vi "Subvi Add Offset to XY Coordinates.vi"(1 "YOffsetIn":i32, 2 "XOffsetIn":i32, 3 "TileXYCoordinatesIn":i32[][](array[numeric])) -> (0 "TileXYCoordinatesOut":i32[][](array[numeric]))   [LabVIEW 2012]
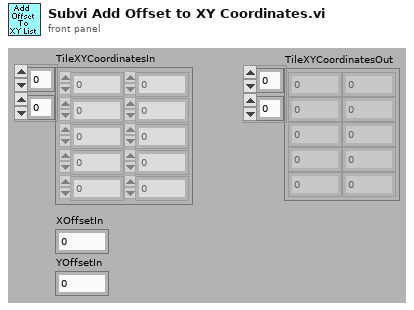
[diagram p1: front panel]
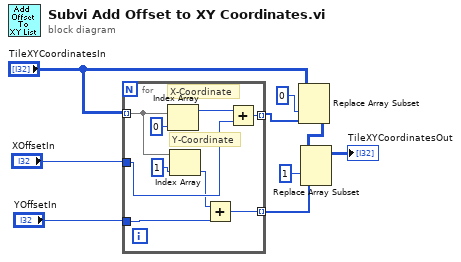
[diagram p0: block diagram]
diagram:
  n1 = for {
    tunnel: "TileXYCoordinatesIn" -> [w16] mode=indexing
    tunnel: "XOffsetIn" -> [w14]
    tunnel: "YOffsetIn" -> [w12]
    tunnel: [w11] -> w8 mode=indexing
    tunnel: [w10] -> w6 mode=indexing
    # "Y-Coordinate"
    # "X-Coordinate"
    n2 = Index Array(array=w16, index=0) -> (element=w15:i32)
    n3 = Index Array(array=w16, index=1) -> (element=w13:i32)
    n4 = Add(x=w13, y=w12) -> (x+y=w10:i32)
    n5 = Add(x=w15, y=w14) -> (x+y=w11:i32)
  }
  n6 = Replace Array Subset(array="TileXYCoordinatesIn", new element=w8, index (col)=0 ("disabled index (col)")) -> (w5:i32[][])  [unwired: 1 in]
  n7 = Replace Array Subset(array=w5, new element=w6, index (col)=1 ("disabled index (col)")) -> (→"TileXYCoordinatesOut":i32[][])  [unwired: 1 in]
